vi "Main.vi"() -> ()   [LabVIEW 2020, in "SubPanels.lvlib"]
uses:
  SubPanels.lvlib
  OOPanel/Manager/Manager.lvclass
  SubClone/SubClone.lvclass
panel:
  in  "X A":bool
  in  "Out A":bool
  in  "X B":bool
  in  "Out B":bool
  in  "Y - B":bool
  in  "Y - A":bool
  in  "G - B":bool
  in  "G - A":bool
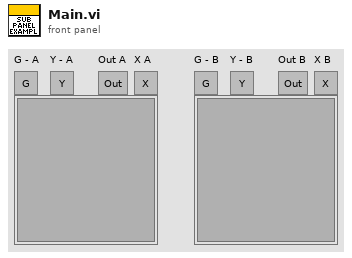
[diagram p1: front panel]
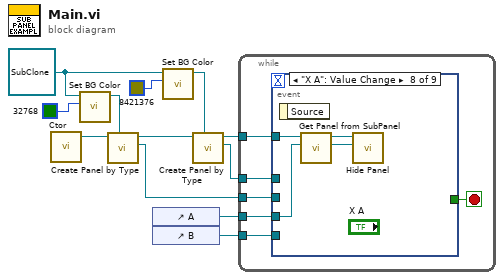
[diagram p0: block diagram]
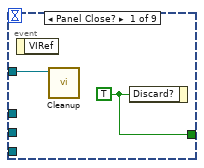
[diagram p2: hidden frame]
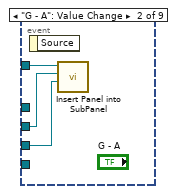
[diagram p3: hidden frame]
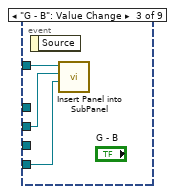
[diagram p4: hidden frame]
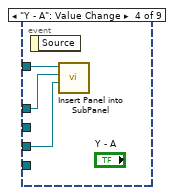
[diagram p5: hidden frame]
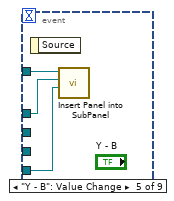
[diagram p6: hidden frame]
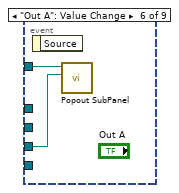
[diagram p7: hidden frame]
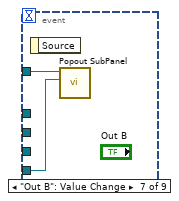
[diagram p8: hidden frame]
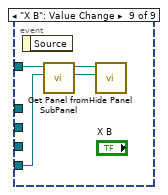
[diagram p9: hidden frame]
diagram:
  w1 = refnum<class "SubClone.lvclass"> refnum ("SubPanels.lvlib:SubClone.lvclass")
  n1 = call "Ctor.vi"() -> ("Manager out"=w9:refnum<class "Manager.lvclass">)  [unwired: 10 in, 1 out]
  n2 = call "Set BG Color.vi"("BG"=u32 32768, "SubClone in"=w1) -> ("SubClone out"=w10:refnum<class "SubClone.lvclass">)  [unwired: 8 in, 1 out]
  n3 = call "Create Panel by Type.vi"("Panel Type"=w10, "Manager in"=w9) -> ("Panel"=w3:refnum<class "SubClone.lvclass">, "Manager out"=w8:refnum<class "Manager.lvclass">)  [unwired: 7 in, 1 out]
  n4 = control-ref of="A"() -> (w5:refnum<vi>)
  n5 = control-ref of="B"() -> (w4:refnum<vi>)
  n6 = call "Set BG Color.vi"("BG"=u32 8421376, "SubClone in"=w1) -> ("SubClone out"=w7:refnum<class "SubClone.lvclass">)  [unwired: 8 in, 1 out]
  n7 = call "Create Panel by Type.vi"("Panel Type"=w7, "Manager in"=w8) -> ("Panel"=w2:refnum<class "SubClone.lvclass">, "Manager out"=w6:refnum<class "Manager.lvclass">)  [unwired: 7 in, 1 out]
  n8 = while {
    tunnel: w6 -> [w18]
    tunnel: w5 -> [w17]
    tunnel: w4 -> [w16]
    tunnel: w3 -> [w14]
    tunnel: w2 -> [w13]
    stop <- w15 stop-if-true
    n9 = event shown="[7] \"X A\": Value Change" {
      selector: _ -> [_ _ _ _ _ _ _ _ _]
      dyn-events: _ -> [_ _ _ _ _ _ _ _ _]
      timeout: _ -> [_ _ _ _ _ _ _ _ _]
      tunnel: w18 -> [w19 w23 w26 w29 w32 w34 w36 w40 w44]
      tunnel: w17 -> [_ w21 _ w27 _ w33 _ w39 _]
      tunnel: w16 -> [_ _ w24 _ w31 _ w35 _ w41]
      tunnel: [w20 _ _ _ _ _ _ _ _] -> w15
      tunnel: w14 -> [_ w22 w25 _ _ _ _ _ _]
      tunnel: w13 -> [_ _ _ w28 w30 _ _ _ _]
      event Panel Close? {
        w20 = TRUE ("Discard?")
        n10 = event-data() -> ()  [unwired: 1 in, 1 out]
        n11 = call "Cleanup.vi"("Manager in"=w19) -> ()  [unwired: 8 in, 3 out]
        n12 = event-data("Discard?"=w20) -> ()  [unwired: 1 in, 1 out]
      }
      event "G - A": Value Change {
        n13 = event-data() -> ()  [unwired: 1 in, 1 out]
        n14 = call "Insert Panel into SubPanel.vi"("SubPanel"=w21, "Panel In"=w22, "Manager in"=w23) -> ()  [unwired: 6 in, 3 out]
      }
      event "G - B": Value Change {
        n15 = event-data() -> ()  [unwired: 1 in, 1 out]
        n16 = call "Insert Panel into SubPanel.vi"("SubPanel"=w24, "Panel In"=w25, "Manager in"=w26) -> ()  [unwired: 6 in, 3 out]
      }
      event "Y - A": Value Change {
        n17 = event-data() -> ()  [unwired: 1 in, 1 out]
        n18 = call "Insert Panel into SubPanel.vi"("SubPanel"=w27, "Panel In"=w28, "Manager in"=w29) -> ()  [unwired: 6 in, 3 out]
      }
      event "Y - B": Value Change {
        n19 = event-data() -> ()  [unwired: 1 in, 1 out]
        n20 = call "Insert Panel into SubPanel.vi"("SubPanel"=w31, "Panel In"=w30, "Manager in"=w32) -> ()  [unwired: 6 in, 3 out]
      }
      event "Out A": Value Change {
        n21 = event-data() -> ()  [unwired: 1 in, 1 out]
        n22 = call "Popout SubPanel.vi"("SubPanel"=w33, "Manager in"=w34) -> ()  [unwired: 8 in, 2 out]
      }
      event "Out B": Value Change {
        n23 = event-data() -> ()  [unwired: 1 in, 1 out]
        n24 = call "Popout SubPanel.vi"("SubPanel"=w35, "Manager in"=w36) -> ()  [unwired: 8 in, 2 out]
      }
      event "X A": Value Change {
        n25 = event-data() -> ()  [unwired: 1 in, 1 out]
        n26 = call "Get Panel from SubPanel.vi"("SubPanel"=w39, "Manager in"=w40) -> ("Panel"=w37:refnum<class "Panel.lvclass">, "Manager out"=w38:refnum<class "Manager.lvclass">)  [unwired: 6 in, 2 out]
        n27 = call "Hide Panel.vi"("Panel In"=w37, "Manager in"=w38) -> ()  [unwired: 7 in, 3 out]
      }
      event "X B": Value Change {
        n28 = event-data() -> ()  [unwired: 1 in, 1 out]
        n29 = call "Get Panel from SubPanel.vi"("SubPanel"=w41, "Manager in"=w44) -> ("Panel"=w42:refnum<class "Panel.lvclass">, "Manager out"=w43:refnum<class "Manager.lvclass">)  [unwired: 6 in, 2 out]
        n30 = call "Hide Panel.vi"("Panel In"=w42, "Manager in"=w43) -> ()  [unwired: 7 in, 3 out]
      }
    }
  }
